vi "8-bit video export-AVI write by mode.vi"(8 "error in (no error)":errorcluster, 10 "RGB image ref in":T4, 11 "AVI modes refs":T1) -> (0 "error out":errorcluster, 3 "AVI modes refs":T1)   [LabVIEW 2020]
uses:
  <vilib>/vision/Image Controls.llb/IMAQ Image.ctl
  Typedefs/8-bit video export AVI modes cluster.ctl
  <vilib>/vision/Avi1.llb/AviRefnum.ctl
  <vilib>/vision/Avi.llb/IMAQ AVI2 Refnum.ctl
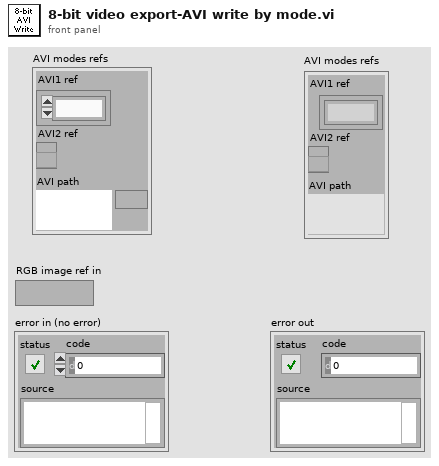
[diagram p1: front panel]
types:
  T1 = typedef "8-bit video export AVI modes cluster.ctl" = cluster{"AVI1 ref":T2, "AVI2 ref":T3, "AVI path":path}
  T2 = typedef "AviRefnum.ctl" = refnum<k1>
  T3 = typedef "IMAQ AVI2 Refnum.ctl" = refnum<k20>
  T4 = typedef "IMAQ Image.ctl" = refnum<image>
  T5 = typedef "AVI implementation enum.ctl" = enum16{"AVI1", "AVI2"}
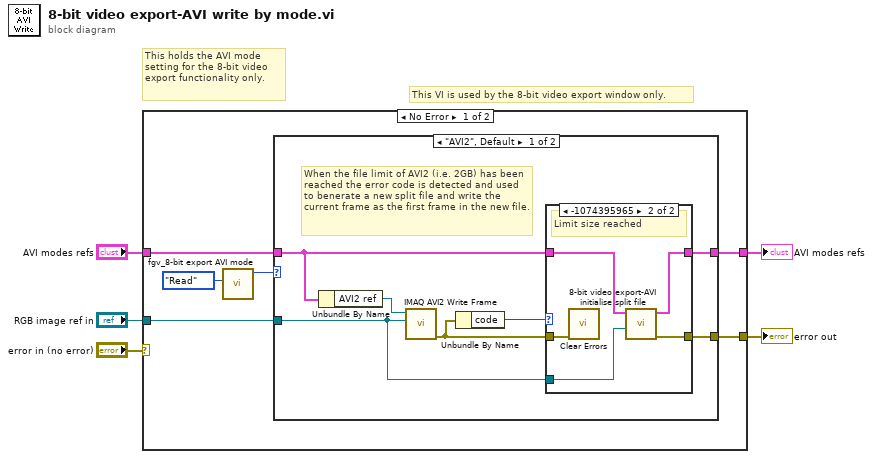
[diagram p0: block diagram]
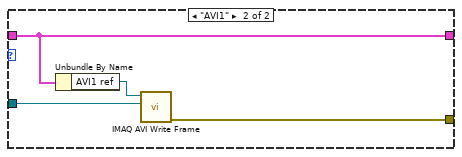
[diagram p3: hidden frame]
diagram:
  # "This VI is used by the 8-bit video export window only."
  # "This holds the AVI mode setting for the 8-bit video export functionality only."
  n1 = case shown="No Error" "error in (no error)" {
    selector: "error in (no error)" -> [_ w31]
    tunnel: "RGB image ref in" -> [w11 _]
    tunnel: "AVI modes refs" -> [w10 w30]
    tunnel: [w9 w30] -> w3
    tunnel: [w8 w31] -> w2
    frame No Error {
      n2 = call "fgv_8-bit export AVI mode.vi"("Function"=enum16{"Intialize", "Write", "Read", "Clear"}."Read") -> ("AVI mode"=w6:T5)  [unwired: 9 in, 1 out]
      n3 = case shown="\"AVI2\", Default" w6 {
        tunnel: [w17 w27] -> w8
        tunnel: w10 -> [w16 w29]
        tunnel: w11 -> [w12 w26]
        tunnel: [w15 w29] -> w9
        frame "AVI2", Default {
          # "When the file limit of AVI2 (i.e. 2GB) has been reached the error code is detected and used to benerate a new split file and write the current frame as the first frame in the new file."
          n4 = Unbundle By Name(w16) -> ("AVI2 ref"=w18:T3)
          n5 = call "IMAQ AVI2 Write Frame"("Image"=w12, "AVI Refnum"=w18) -> ("error out"=w14:errorcluster)  [unwired: 7 in, 2 out]
          n6 = Unbundle By Name(w14) -> ("code"=w13:i32)
          n7 = case shown="-1074395965" w13 {
            tunnel: w14 -> [w20 w22]
            tunnel: [w20 w25] -> w17
            tunnel: w16 -> [w19 w24]
            tunnel: [w19 w23] -> w15
            tunnel: w12 -> [_ w21]
            frame Default {
              # "2GB limit not reached yet"
            }
            frame -1074395965 {
              # "Limit size reached"
              n8 = call <vilib>:"Clear Errors.vi"("error in (no error)"=w22) -> ()  [unwired: 5 in, 2 out]
              n9 = call "8-bit video export-AVI initialise split file.vi"("RGB image ref in"=w21, "AVI modes refs"=w24) -> ("error out"=w25:errorcluster, "AVI modes refs"=w23:T1)  [unwired: 8 in]
            }
          }
        }
        frame "AVI1" {
          n10 = Unbundle By Name(w29) -> ("AVI1 ref"=w28:T2)
          n11 = call "IMAQ AVI Write Frame"("Image"=w26, "Avi Refnum"=w28) -> ("error out"=w27:errorcluster)  [unwired: 8 in, 1 out]
        }
      }
    }
    frame Error {
    }
  }
  "error out" <- w2
  "AVI modes refs" <- w3
